vi "AK8963 meg offset.vi"(1 "measure":dbl[](array[numeric])) -> (0 "measure OUT":dbl[](array[numeric]))   [LabVIEW 2019]
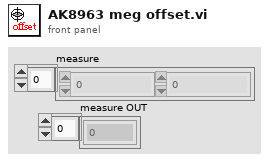
[diagram p1: front panel]
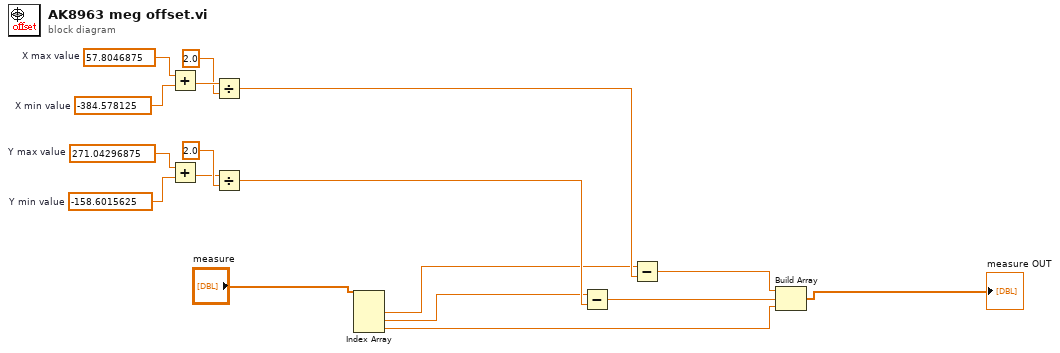
[diagram p0: block diagram]
diagram:
  w16 = 57.8046875  # X max value
  w17 = -384.578125  # X min value
  w11 = 271.04296875  # Y max value
  w10 = -158.6015625  # Y min value
  n1 = Add(x=w16, y=w17) -> (x+y=w15:dbl)
  n2 = Add(x=w11, y=w10) -> (x+y=w12:dbl)
  n3 = Divide(x=w15, y=2.0) -> (x/y=w8:dbl)
  n4 = Divide(x=w12, y=2.0) -> (x/y=w7:dbl)
  n5 = Index Array(array="measure") -> (element #1=w6:dbl, element #2=w5:dbl, element #3=w2:dbl)  [unwired: 3 in]
  n6 = Subtract(x=w5, y=w7) -> (x-y=w3:dbl)
  n7 = Subtract(x=w6, y=w8) -> (x-y=w4:dbl)
  n8 = Build Array(w4, w3, w2) -> (→"measure OUT":dbl[])
